vi "JSON to UTF8 String.vi"(9 "error in (no error)":errorcluster, 10 "Offset":i32, 11 "JSON":string) -> (1 "error out":errorcluster, 3 "<UTF8>String":string)   [LabVIEW 2021, in "json.facade.lvlib"]
doc: "Convert JSON to a UTF-8 encoded String."
uses:
  json.facade.lvlib
  jsontext/JSONtext.lvlib
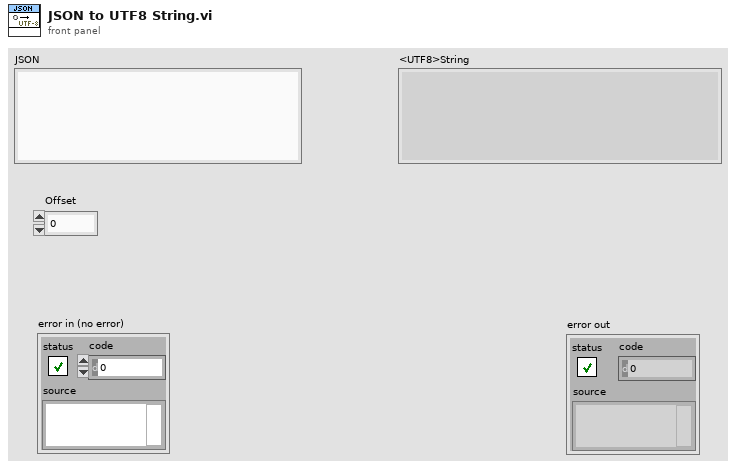
[diagram p1: front panel]
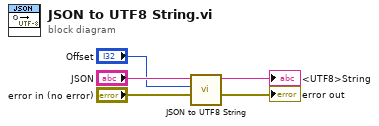
[diagram p0: block diagram]
diagram:
  n1 = call "JSON to UTF8 String.vi"("error in (no error)"="error in (no error)", "Offset"="Offset", "JSON"="JSON") -> ("error out"=→"error out":errorcluster, "<UTF8>String"=→"<UTF8>String":string)  [unwired: 7 in]
